vi "Initialize Instrument.vi"(8 "error in (no error)":errorcluster, 10 "Reset":bool, 11 "Agilent 6xxx in":refnum<class "Agilent 6xxx.lvclass">) -> (0 "error out":errorcluster, 3 "Agilent 6xxx out":refnum<class "Agilent 6xxx.lvclass">)   [LabVIEW 2020, in "Agilent 6xxx.lvclass"]
uses:
  Agilent 6xxx.lvclass
  C:/Sandbox/RF Bench/Source Code/WiSpry Test Framework/Instruments/Instrument.lvclass
  C:/Sandbox/RF Bench/Source Code/WiSpry Test Framework/Instruments/Power Supply/Power Supply.lvclass
  Power Supply.lvclass/Power Supply.ctl
  Instrument.lvclass/Instrument.ctl
  Instrument.lvclass
  <instrlib>/Agilent 6XXX Series/Agilent 6XXX Series.lvlib
  Power Supply.lvclass
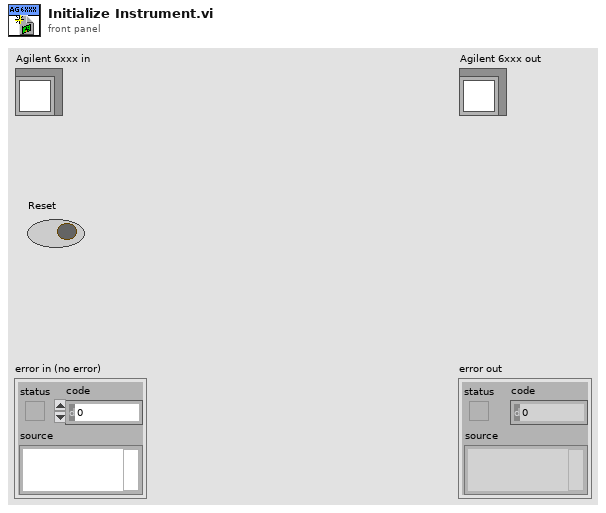
[diagram p1: front panel]
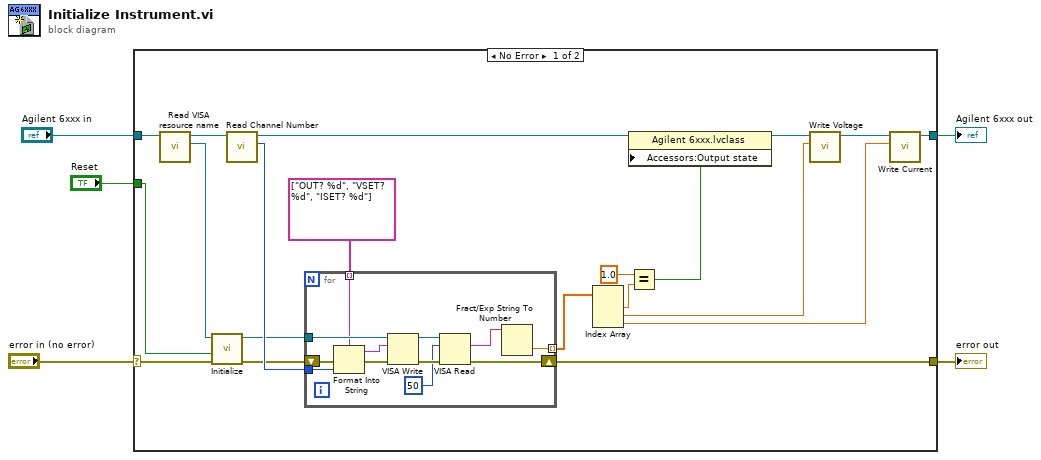
[diagram p0: block diagram]
diagram:
  n1 = case shown="No Error" "error in (no error)" {
    selector: "error in (no error)" -> [w24 w39]
    tunnel: [w20 w39] -> w4
    tunnel: [w7 w38] -> w3
    tunnel: "Agilent 6xxx in" -> [w25 w38]
    tunnel: "Reset" -> [w17 _]
    frame No Error {
      n2 = call "Read VISA resource name.vi"("Instrument in"=w25) -> ("VISA resource name"=w23:refnum<visa-resource-name>, "Instrument out"=w22:refnum<class "Agilent 6xxx.lvclass">)  [unwired: 9 in]
      n3 = call <instrlib>:"Initialize.vi"("error in (no error)"=w24, "Reset (T: Reset)"=w17, "VISA resource name"=w23) -> ("error out"=w18:errorcluster, "VISA resource name out"=w19:refnum<visa-resource-name>)  [unwired: 7 in]
      n4 = call "Read Channel Number.vi"("Power Supply in"=w22) -> ("Channel Number"=w21:u8, "Power Supply out"=w8:refnum<class "Agilent 6xxx.lvclass">)  [unwired: 9 in]
      n5 = for {
        tunnel: w21 -> [w37]
        tunnel: w19 -> [w32]
        shift-right: [w34] -> w20
        shift-left: w18 -> [w31]
        tunnel: string[] ["OUT? %d", "VSET? %d", "ISET? %d"] -> [w28] mode=indexing
        tunnel: [w26] -> w15 mode=indexing
        n6 = Format Into String(format string=w28, error in=w31, w37) -> (resulting string=w36:string, error out=w30:errorcluster)  [unwired: 1 in]
        n7 = VISA Write(VISA resource name=w32, write buffer=w36, error in (no error)=w30) -> (VISA resource name out=w33:refnum<visa-resource-name>, error out=w35:errorcluster)  [unwired: 1 out]
        n8 = VISA Read(VISA resource name=w33, byte count=u32 50, error in (no error)=w35) -> (read buffer=w27:string, error out=w34:errorcluster)  [unwired: 2 out]
        n9 = Fract/Exp String To Number(string=w27) -> (number=w26:dbl)  [unwired: 3 in, 1 out]
      }
      n10 = Index Array(array=w15) -> (element #1=w14:dbl, element #2=w12:dbl, element #3=w11:dbl)  [unwired: 3 in]
      n11 = Equal?(x=1.0, y=w14) -> (x = y?=w6:bool)
      n12 = property class="Agilent 6xxx.lvclass"(reference=w8, "Accessors:Output state"=w6) -> (reference out=w10:refnum<class "Agilent 6xxx.lvclass">)  [unwired: 1 in, 1 out]
      n13 = call "Write Voltage.vi"("Voltage"=w12, "Power Supply in"=w10) -> ("Power Supply out"=w9:refnum<class "Agilent 6xxx.lvclass">)  [unwired: 9 in]
      n14 = call "Write Current.vi"("Current"=w11, "Power Supply in"=w9) -> ("Power Supply out"=w7:refnum<class "Agilent 6xxx.lvclass">)  [unwired: 9 in]
    }
    frame Error {
    }
  }
  "error out" <- w4
  "Agilent 6xxx out" <- w3
